vi "BRIF.vi"() -> ()   [LabVIEW 2018]
uses:
  <vilib>/MakerHub/LINX/Public/Peripherals/Digital/Digital Write 1 Chan.vi
  <vilib>/MakerHub/LINX/Public/Peripherals/Digital/Digital Write N Chans.vi
  <vilib>/MakerHub/LINX/Private/Local IO/LinxDigitalWrite.vi
  <vilib>/MakerHub/LINX/Public/Utilities/Check Channel.vi
  <vilib>/MakerHub/LINX/Public/Utilities/Open Serial.vi
  <vilib>/MakerHub/LINX/Private/Utilties/Generate Error.vi
  <vilib>/MakerHub/LINX/LMH-LINX.lvlib
panel:
  in  "Tab Control":enum32{"Initialization", "Calculation"}(tab)
  in  "Serial Port":refnum<visa-resource-name>
  out "Time (ms)":dbl
  in  "Hold \nat Stressed\n(ms)":u16=500 min=500 step=10
  in  "Freq":u16=13 step=100
  in  "Hold \nat Flexed\n(ms)":u16=500 step=10
  in  "Hold \nat Rest after Flexed\n(ms)":u16=500 step=10
  in  "Hold\nat Rest after Stressed\n(ms)":u16=500 step=10
  in  "Cycles":u16=13 step=10
  in  "Stretch\nCourse (mm)":u16=13 step=1
  in  "Flex\nCourse (mm)":u16=13 step=1
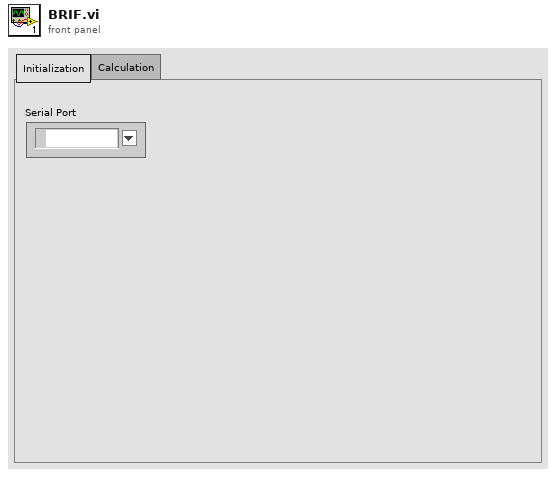
[diagram p1: front panel]
types:
  T1 = typedef "LMH-LINX.lvlib/LINX Ref.ctl" = cluster{"IO":T2, "Interface":T3, "LINX Device Config":T4}
  T2 = typedef "LMH-LINX.lvlib/Platform.ctl" = enum16{"Remote", "Local"}
  T3 = typedef "LMH-LINX.lvlib/Interface.ctl" = enum16{"Serial", "TCP"}
  T4 = typedef "LMH-LINX.lvlib/Device.lvlib/LINX Device Config.ctl" = cluster{"Interface":T3, "COM Port":refnum<visa-resource-name>, "TCP Configuration":T5, "Device Family":u8, "Device ID":u8, "Device Name":string, "TCP Ref":refnum<k5>, "Channels":T6}
  T5 = typedef "LMH-LINX.lvlib/Device.lvlib/TCP Config.ctl" = cluster{"IP Address":string, "Port":u16}
  T6 = typedef "LMH-LINX.lvlib/Channels.ctl" = cluster{"DI":u8[], "DO":u8[], "AI":u8[], "AO":u8[], "PWM":u8[], "QE":u8[], "UART":u8[], "I2C 2":u8[], "SPI":u8[], "CAN":u8[], "Servo":u8[], "AI Ref (V)":dbl, "AI Resolution (Bits)":u8, "AO Ref (V)":dbl, "AO Resolution (Bits)":u8}
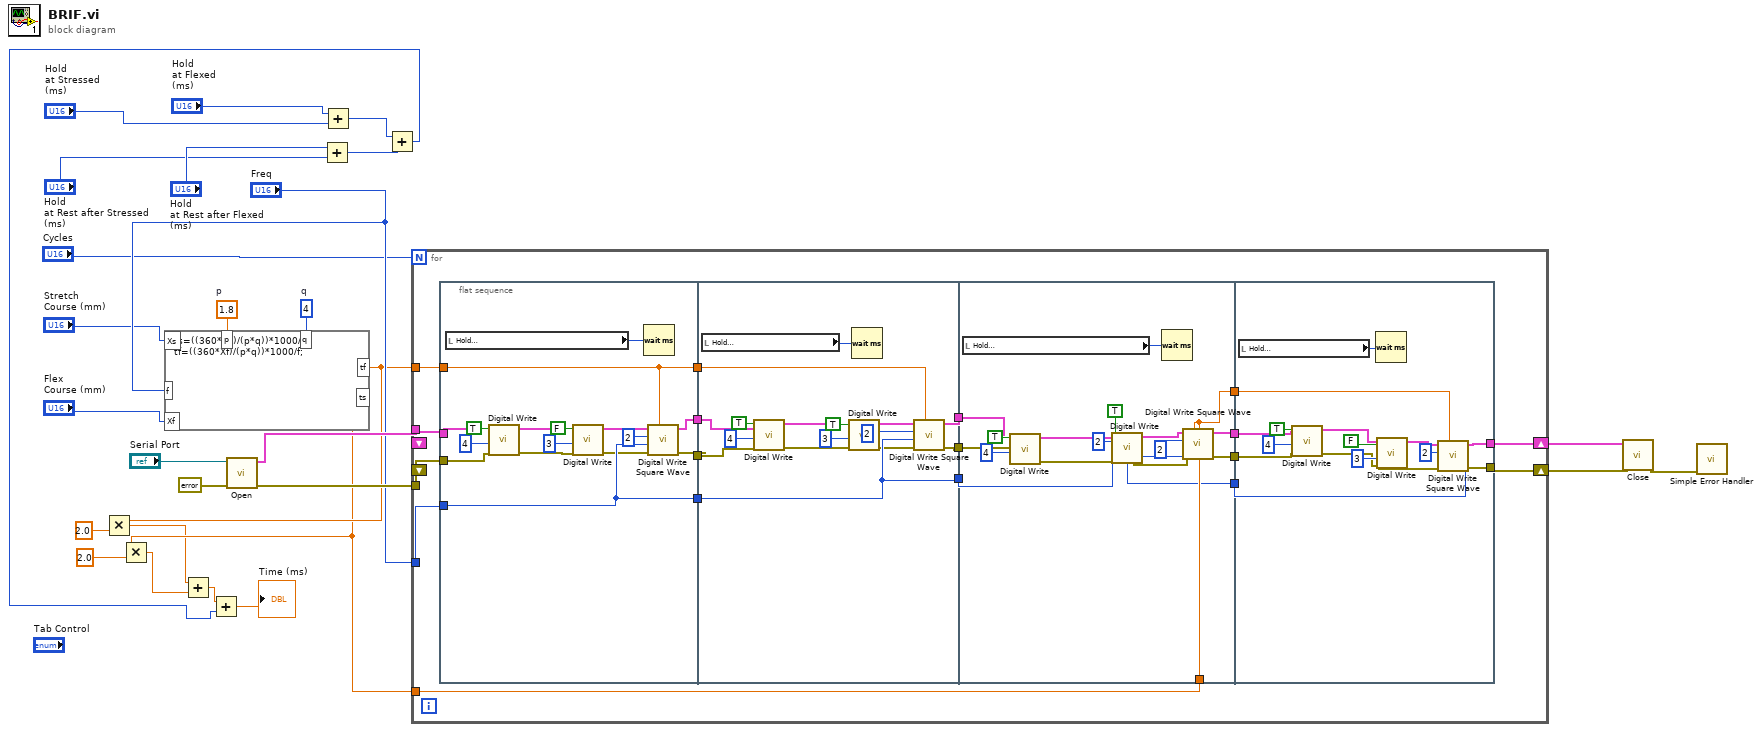
[diagram p0: block diagram]
diagram:
  w27 = 4  # q
  w28 = 1.8  # p
  n1 = formula code="ts=((360*Xs)/(p*q))*1000/f;\ntf=((360*Xf)/(p*q))*1000/f;"("p"=w28, "q"=w27, "Xs"="Stretch\nCourse (mm)", "Xf"="Flex\nCourse (mm)", "f"="Freq") -> ("tf"=w13:dbl, "ts"=w12:dbl)
  n2 = Multiply(x=w13, y=2.0) -> (x*y=w10:dbl)
  n3 = Multiply(x=w12, y=2.0) -> (x*y=w11:dbl)
  n4 = Add(x=w10, y=w11) -> (x+y=w9:dbl)
  n5 = call-poly <vilib>:"Open.vi"("Error In"=errorcluster {"status"=FALSE, "code"=0, "source"=""}, "Serial Port"="Serial Port") -> ("Error Out"=w24:errorcluster, "LINX Resource"=w25:T1)  [unwired: 7 in, 1 out]
  n6 = Add(x="Hold \nat Rest after Flexed\n(ms)", y="Hold\nat Rest after Stressed\n(ms)") -> (x+y=w3:u16)
  n7 = Add(x="Hold \nat Flexed\n(ms)", y="Hold \nat Stressed\n(ms)") -> (x+y=w4:u16)
  n8 = Add(x=w4, y=w3) -> (x+y=w2:u16)
  n9 = Add(x=w9, y=w2) -> (x+y=→"Time (ms)":dbl)
  n10 = for {
    N: "Cycles" -> [_]
    tunnel: w25 -> [w46]
    tunnel: w24 -> [w45]
    tunnel: "Freq" -> [w44]
    tunnel: w13 -> [w43]
    tunnel: w12 -> [w35]
    shift-right: [w30] -> w21
    shift-left: _ -> [_]
    shift-right: [w29] -> w20
    shift-left: _ -> [_]
    n11 = flat-sequence {
      tunnel: w46 -> [w50]
      tunnel: w45 -> [w49]
      tunnel: w44 -> [w60]
      tunnel: w43 -> [w57]
      tunnel: [w60] -> w42
      tunnel: [w59] -> w41
      tunnel: [w58] -> w40
      tunnel: [w57] -> w39
      tunnel: w42 -> [w74]
      tunnel: w41 -> [w65]
      tunnel: w40 -> [w66]
      tunnel: w39 -> [w76]
      tunnel: [w75] -> w38
      tunnel: [w74] -> w37
      tunnel: [w73] -> w36
      tunnel: w38 -> [w81]
      tunnel: w37 -> [w91]
      tunnel: w36 -> [w82]
      tunnel: w35 -> [w92]
      tunnel: [w92] -> w34
      tunnel: [w89] -> w33
      tunnel: [w88] -> w32
      tunnel: [w91] -> w31
      tunnel: w34 -> [w108]
      tunnel: w33 -> [w98]
      tunnel: w32 -> [w97]
      tunnel: w31 -> [w107]
      tunnel: [w106] -> w30
      tunnel: [w105] -> w29
      frame #0 {
        n12 = local read "Hold \nat Rest after Flexed\n(ms)"() -> (w62:u16)
        n13 = call-poly <vilib>:"Digital Write.vi"("Error In"=w49, "Output Value"=TRUE, "DO Channel"=u8 4, "LINX Resource"=w50) -> ("Error Out"=w47:errorcluster, "LINX Resource"=w48:T1)  [unwired: 6 in]
        n14 = call-poly <vilib>:"Digital Write.vi"("Error In"=w47, "Output Value"=FALSE, "DO Channel"=u8 3, "LINX Resource"=w48) -> ("Error Out"=w55:errorcluster, "LINX Resource"=w56:T1)  [unwired: 6 in]
        n15 = Wait (ms)(milliseconds to wait=w62) -> ()  [unwired: 1 out]
        n16 = call <vilib>:"Digital Write Square Wave.vi"("Duration (ms)"=w57, "Error In"=w55, "Frequency (Hz)"=w60, "Channel"=u8 2, "LINX Resource"=w56) -> ("Error Out"=w59:errorcluster, "LINX Resource"=w58:T1)  [unwired: 5 in]
      }
      frame #1 {
        n17 = local read "Hold \nat Stressed\n(ms)"() -> (w78:u16)
        n18 = call-poly <vilib>:"Digital Write.vi"("Error In"=w65, "Output Value"=TRUE, "DO Channel"=u8 4, "LINX Resource"=w66) -> ("Error Out"=w63:errorcluster, "LINX Resource"=w64:T1)  [unwired: 6 in]
        n19 = call-poly <vilib>:"Digital Write.vi"("Error In"=w63, "Output Value"=TRUE, "DO Channel"=u8 3, "LINX Resource"=w64) -> ("Error Out"=w70:errorcluster, "LINX Resource"=w71:T1)  [unwired: 6 in]
        n20 = Wait (ms)(milliseconds to wait=w78) -> ()  [unwired: 1 out]
        n21 = call <vilib>:"Digital Write Square Wave.vi"("Duration (ms)"=w76, "Error In"=w70, "Frequency (Hz)"=w74, "Channel"=u8 2, "LINX Resource"=w71) -> ("Error Out"=w75:errorcluster, "LINX Resource"=w73:T1)  [unwired: 5 in]
      }
      frame #2 {
        n22 = local read "Hold\nat Rest after Stressed\n(ms)"() -> (w94:u16)
        n23 = call-poly <vilib>:"Digital Write.vi"("Error In"=w81, "Output Value"=TRUE, "DO Channel"=u8 4, "LINX Resource"=w82) -> ("Error Out"=w79:errorcluster, "LINX Resource"=w80:T1)  [unwired: 6 in]
        n24 = call-poly <vilib>:"Digital Write.vi"("Error In"=w79, "Output Value"=TRUE, "DO Channel"=u8 2, "LINX Resource"=w80) -> ("Error Out"=w86:errorcluster, "LINX Resource"=w87:T1)  [unwired: 6 in]
        n25 = Wait (ms)(milliseconds to wait=w94) -> ()  [unwired: 1 out]
        n26 = call <vilib>:"Digital Write Square Wave.vi"("Duration (ms)"=w92, "Error In"=w86, "Frequency (Hz)"=w91, "Channel"=u8 2, "LINX Resource"=w87) -> ("Error Out"=w88:errorcluster, "LINX Resource"=w89:T1)  [unwired: 5 in]
      }
      frame #3 {
        n27 = local read "Hold \nat Flexed\n(ms)"() -> (w110:u16)
        n28 = call-poly <vilib>:"Digital Write.vi"("Error In"=w97, "Output Value"=TRUE, "DO Channel"=u8 4, "LINX Resource"=w98) -> ("Error Out"=w95:errorcluster, "LINX Resource"=w96:T1)  [unwired: 6 in]
        n29 = Wait (ms)(milliseconds to wait=w110) -> ()  [unwired: 1 out]
        n30 = call-poly <vilib>:"Digital Write.vi"("Error In"=w95, "Output Value"=FALSE, "DO Channel"=u8 3, "LINX Resource"=w96) -> ("Error Out"=w102:errorcluster, "LINX Resource"=w103:T1)  [unwired: 6 in]
        n31 = call <vilib>:"Digital Write Square Wave.vi"("Duration (ms)"=w108, "Error In"=w102, "Frequency (Hz)"=w107, "Channel"=u8 2, "LINX Resource"=w103) -> ("Error Out"=w106:errorcluster, "LINX Resource"=w105:T1)  [unwired: 5 in]
      }
    }
  }
  n32 = call <vilib>:"Close.vi"("Error In"=w21, "LINX Resource"=w20) -> ("Error Out"=w22:errorcluster)  [unwired: 9 in]
  n33 = call <vilib>:"Simple Error Handler.vi"("error in (no error)"=w22) -> ()  [unwired: 4 in, 5 out]
